vi "송신.vi"() -> ()   [LabVIEW 2023]
panel:
  in  "Stop Button":bool=TRUE
  in  "Target IP":string
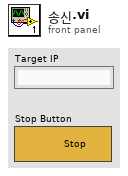
[diagram p1: front panel]
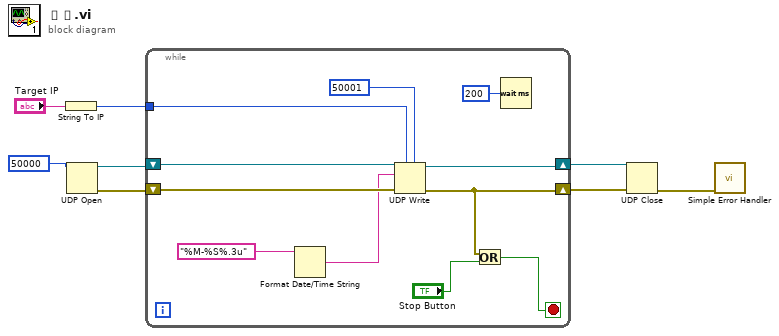
[diagram p0: block diagram]
diagram:
  n1 = String To IP(1:"Target IP") -> (0:w4:u32)
  n2 = UDP Open(11:u16 50000 ("port")) -> (port=w6:refnum<k16>, 0:w8:errorcluster)  [unwired: 4 in, 1 out]
  n3 = while {
    shift-right: [w17] -> w5
    shift-left: w6 -> [w18]
    shift-right: [w10] -> w7
    shift-left: w8 -> [w19]
    tunnel: w4 -> [w15]
    stop <- w11 stop-if-true
    n4 = Format Date/Time String(time format string (%c)="%M-%S%.3u") -> (date/time string=w13:string)  [unwired: 2 in]
    n5 = UDP Write(address=w15, port or service name=u16 50001, connection ID=w18, data in=w13, 8:w19) -> (error out=w10:errorcluster, 3:w17:refnum<k16>)  [unwired: 1 in]
    n6 = Or(x=w10, y="Stop Button") -> (x .or. y?=w11:bool)
    n7 = Wait (ms)(milliseconds to wait=u32 200) -> ()  [unwired: 1 out]
  }
  n8 = UDP Close(connection ID=w5, 8:w7) -> (error out=w1:errorcluster)  [unwired: 1 out]
  n9 = call <vilib>:"Simple Error Handler.vi"("error in (no error)"=w1) -> ()  [unwired: 4 in, 5 out]
